vi "uDAQwriteCmd.vi"(8 "error in (no error)":errorcluster, 9 "ParamByte":u8, 10 "CmdByte":u8, 11 "connection ID":refnum<k5>) -> (0 "error out":errorcluster, 3 "connection ID out":refnum<k5>)   [LabVIEW 2017]
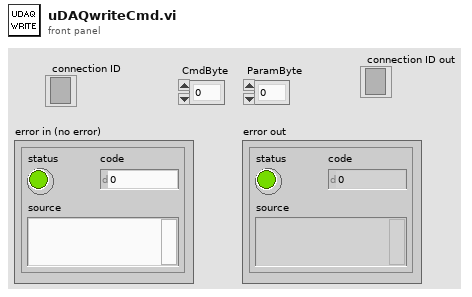
[diagram p1: front panel]
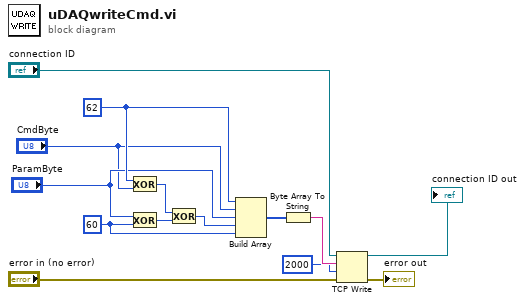
[diagram p0: block diagram]
diagram:
  w13 = u8 60
  w14 = u8 62
  n1 = Exclusive Or(1:"CmdByte", 2:w14) -> (0:w9:u8)
  n2 = Exclusive Or(1:w13, 2:"ParamByte") -> (0:w8:u8)
  n3 = Exclusive Or(1:w8, 2:w9) -> (0:w10:u8)
  n4 = Build Array(w14, "CmdByte", "ParamByte", w10, w13) -> (w12:u8[])
  n5 = Byte Array To String(unsigned byte array=w12) -> (string=w11:string)
  n6 = TCP Write(connection ID="connection ID", data in=w11, error in (no error)="error in (no error)", 9:2000) -> (connection ID out=→"connection ID out":refnum<k5>, error out=→"error out":errorcluster)  [unwired: 1 out]
